vi "Sample Acquisition.vi"(8 "error in (no error)":errorcluster, 9 "Samples per Read":u32, 10 "Channel in":T2, 11 "DeviceRefnum Out in":u64) -> (0 "error out":errorcluster, 2 "Channel out":T1, 3 "DeviceRefnum Out out":u64)   [LabVIEW 2016]
uses:
  <extravilib>/ChannelInstances/Tag-bool/))Channel.ctl
  <extravilib>/ChannelInstances/High Speed Stream-a[.](u8)/)Channel.ctl
  <extravilib>/ChannelInstances/Tag-bool/Read With Abort.vi
  <extravilib>/ChannelInstances/Tag-bool/Endpoint.vi
  <extravilib>/ChannelInstances/High Speed Stream-a[.](u8)/)Channel.vi
  <vilib>/rtlsdr/rtlsdr.lvlib
  <extravilib>/ChannelInstances/High Speed Stream-a[.](u8).lvlib
  <extravilib>/ChannelInstances/Tag-bool.lvlib
panel:
  out "x-y":dbl
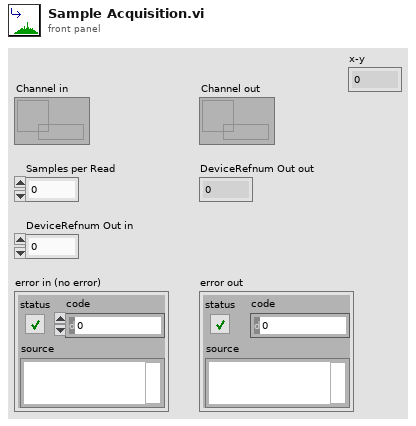
[diagram p1: front panel]
types:
  T1 = typedef "High Speed Stream-a[.](u8).lvlib/)Channel.ctl" = refnum<queue>
  T2 = typedef "Tag-bool.lvlib/))Channel.ctl" = refnum<queue>
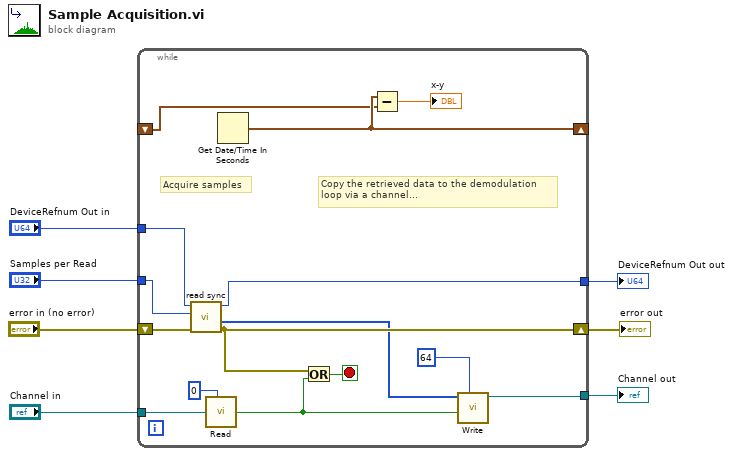
[diagram p0: block diagram]
diagram:
  n1 = while {
    shift-right: [w18] -> w2
    shift-left: "error in (no error)" -> [w21]
    tunnel: "Samples per Read" -> [w19]
    tunnel: [w14] -> w6
    tunnel: "Channel in" -> [w12]
    tunnel: "DeviceRefnum Out in" -> [w22]
    tunnel: [w17] -> w3
    shift-right: [w10] -> _
    shift-left: _ -> [w9]
    stop <- w20 stop-if-true
    # "Copy the retrieved data to the demodulation\nloop via a channel..."
    # "Acquire samples"
    n2 = call <vilib>:"read sync.vi"("error in (no error)"=w21, "Number Of Samples"=w19, "DeviceRefnum"=w22) -> ("error out"=w18:errorcluster, "Sample Buffer"=w16:u8[], "DeviceRefnum Out"=w17:u64)  [unwired: 5 in, 1 out]
    n3 = call <extravilib>:"Read.vi"("channel"=w12, "timeout in ms (0)"=0) -> ("element"=w13:bool)  [unwired: 1 out]
    n4 = Get Date/Time In Seconds() -> (seconds since 1Jan1904=w10:timestamp)
    n5 = Or(x=w18, y=w13) -> (x .or. y?=w20:bool)
    n6 = Subtract(x=w10, y=w9) -> (x-y=→"x-y":dbl)
    n7 = call <extravilib>:"Write.vi"("size (unlimited)"=64, "last element? (F)"=w13, "element"=w16) -> ("channel"=w14:T1)  [unwired: 6 in, 2 out]
  }
  "Channel out" <- w6
  "DeviceRefnum Out out" <- w3
  "error out" <- w2
